vi "GetDigitalFilterControl.vi"(8 "Error In":errorcluster, 11 "Keithley 6485 In":refnum<visa-resource-name>) -> (0 "Error Out":errorcluster, 2 "Digital Filter Control":T1, 3 "Keithley 6485 Out":refnum<visa-resource-name>)   [LabVIEW 2012, in "Keithley-6485.lvlib"]
uses:
  Keithley-6485.lvlib
  Controls/DigitalFilterControl.ctl
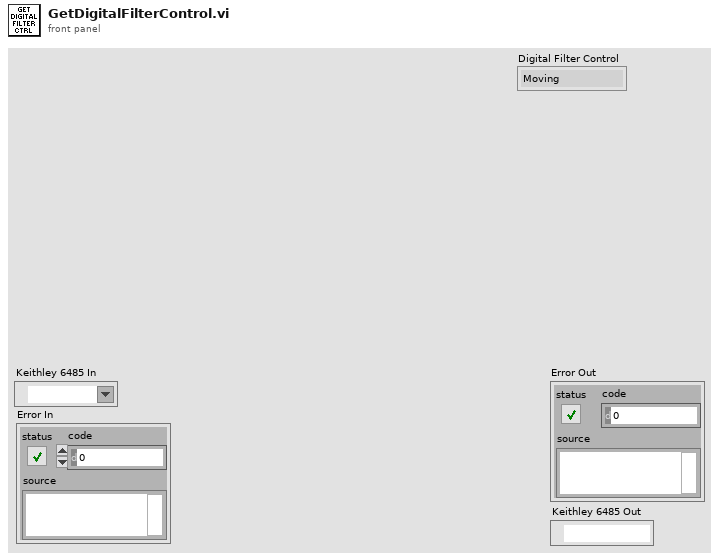
[diagram p1: front panel]
types:
  T1 = typedef "Keithley-6485.lvlib/DigitalFilterControl.ctl" = enum16{"Moving", "Repeat"}
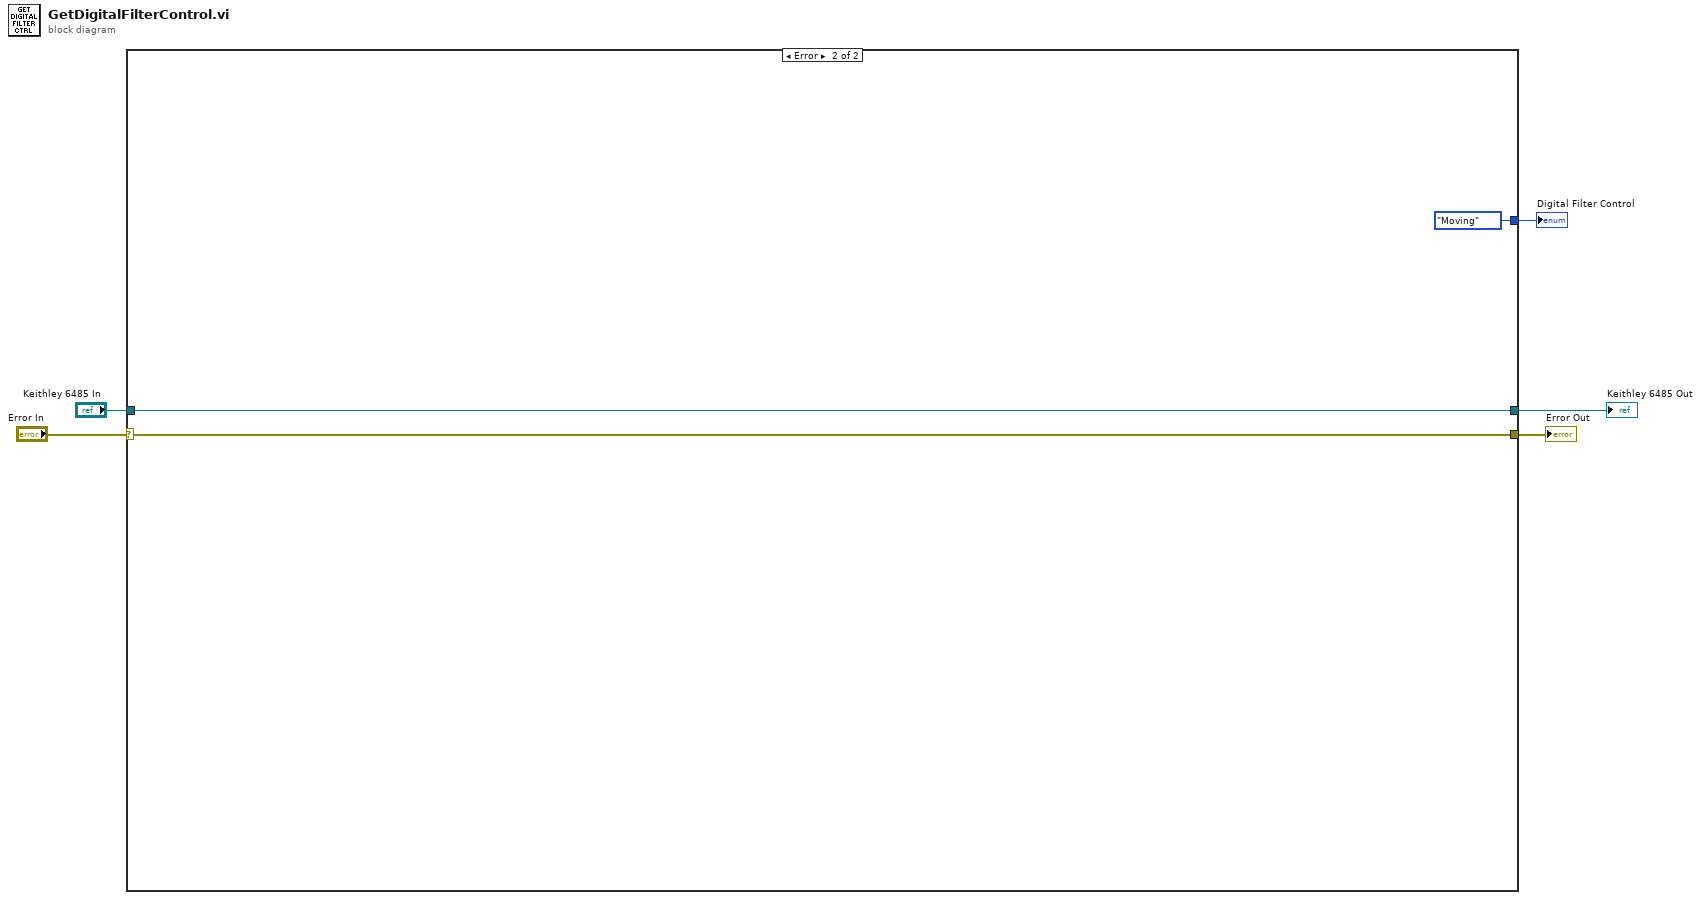
[diagram p0: block diagram]
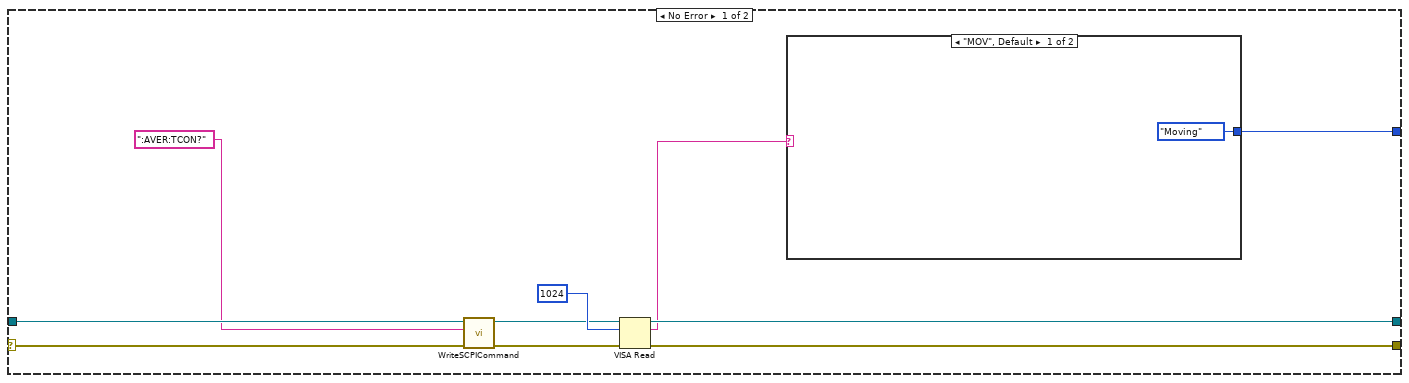
[diagram p2: hidden frame]
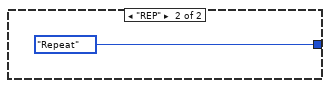
[diagram p3: hidden frame]
diagram:
  n1 = case shown="Error" "Error In" {
    selector: "Error In" -> [w10 w19]
    tunnel: "Keithley 6485 In" -> [w9 w20]
    tunnel: [w15 w19] -> w3
    tunnel: [w14 w20] -> w2
    tunnel: [w6 DigitalFilterControl."Moving" ("Digital Filter Control")] -> w1
    frame No Error {
      n2 = call "WriteSCPICommand.vi"("Error In"=w10, "SCPI Command"=":AVER:TCON?" ("string"), "Keithley 6482 In"=w9) -> ("Error Out"=w11:errorcluster, "Keithley 6482 Out"=w12:refnum<visa-resource-name>)  [unwired: 7 in]
      n3 = VISA Read(VISA resource name=w12, byte count=u32 1024, error in (no error)=w11) -> (VISA resource name out=w14:refnum<visa-resource-name>, read buffer=w8:string, error out=w15:errorcluster)  [unwired: 1 out]
      n4 = case shown="\"MOV\", Default" w8 {
        tunnel: [DigitalFilterControl."Moving" ("Digital Filter Control") DigitalFilterControl."Repeat" ("Digital Filter Control")] -> w6
        frame "MOV", Default {
        }
        frame "REP" {
        }
      }
    }
    frame Error {
    }
  }
  "Error Out" <- w3
  "Keithley 6485 Out" <- w2
  "Digital Filter Control" <- w1
